vi "Copy Built Files.vi"(8 "error in (no error)":errorcluster, 10 "Component Built Path":path, 11 "Repo Built Path":path) -> (0 "error out":errorcluster)   [LabVIEW 2027]
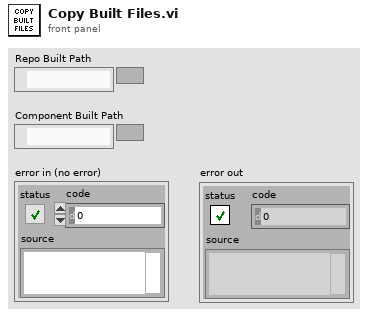
[diagram p1: front panel]
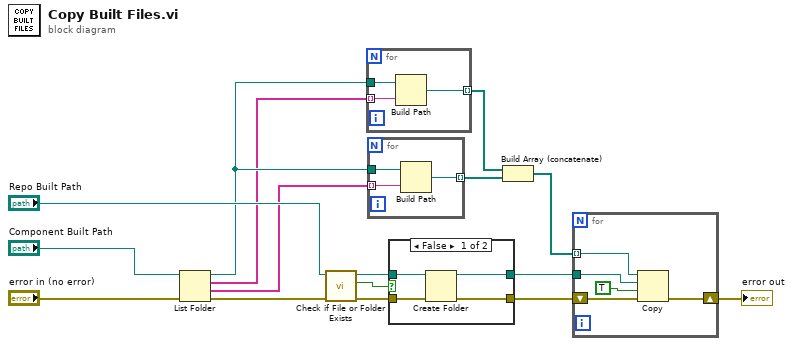
[diagram p0: block diagram]
diagram:
  n1 = List Folder(path="Component Built Path", error in="error in (no error)") -> (path out=w8:path, filenames=w1:string[], folder names=w7:string[], error out=w10:errorcluster)  [unwired: 2 in]
  n2 = call <vilib>:"Check if File or Folder Exists.vi"("error in (no error)"=w10, "path"="Repo Built Path") -> ("error out"=w6:errorcluster, "file or folder exists?"=w4:bool, "dup path"=w5:path)  [unwired: 7 in]
  n3 = for {
    tunnel: w1 -> [w18] mode=indexing
    tunnel: w8 -> [w19]
    tunnel: [w17] -> w2 mode=indexing
    n4 = Build Path(base path=w19, name or relative path=w18) -> (appended path=w17:path)
  }
  n5 = for {
    tunnel: w7 -> [w21] mode=indexing
    tunnel: w8 -> [w22]
    tunnel: [w20] -> w9 mode=indexing
    n6 = Build Path(base path=w22, name or relative path=w21) -> (appended path=w20:path)
  }
  n7 = case shown="False" w4 {
    tunnel: w5 -> [w26 w28]
    tunnel: w6 -> [w25 w27]
    tunnel: [w24 w28] -> w11
    tunnel: [w23 w27] -> w12
    frame False {
      n8 = Create Folder(path (use dialog)=w26, error in=w25) -> (created path=w24:path, error out=w23:errorcluster)  [unwired: 1 in, 1 out]
    }
    frame True {
    }
  }
  n9 = Build Array (concatenate)(w2, w9) -> (w3:path[])
  n10 = for {
    tunnel: w3 -> [w30] mode=indexing
    shift-right: [w31] -> w14
    shift-left: w12 -> [w32]
    tunnel: w11 -> [w29]
    n11 = Copy(8:w32, 9:TRUE ("overwrite (F)"), 10:w29, 11:w30) -> (0:w31:errorcluster)  [unwired: 1 in, 2 out]
  }
  "error out" <- w14
